vi "car coordinate move position in out.vi"(7 "Position in 2":T1, 8 "error in (no error)":errorcluster, 9 "Position in":T1, 11 "move":cluster{"X":dbl, "Y":dbl}) -> (0 "error out":errorcluster, 1 "Position out":T1)   [LabVIEW 2019]
uses:
  move/position cluster.ctl
  V A J control/move cluster(VAJ).ctl
panel:
  out "x+y":dbl
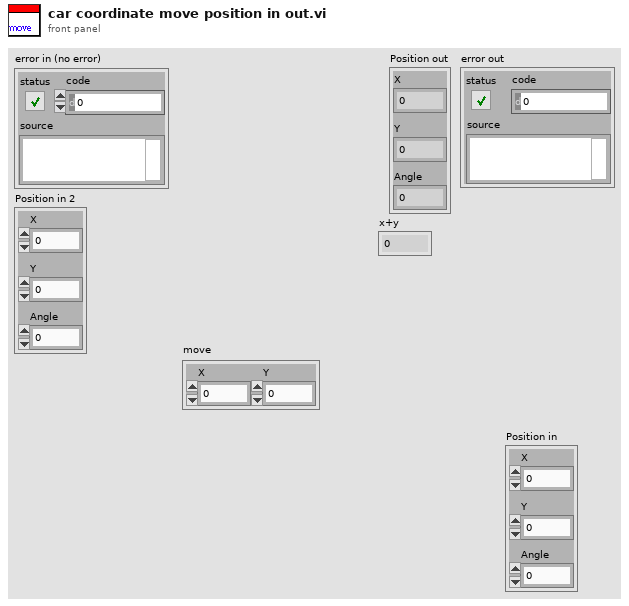
[diagram p1: front panel]
types:
  T1 = typedef "position cluster.ctl" = cluster{"X":dbl, "Y":dbl, "Angle":dbl}
  T2 = typedef "move cluster(VAJ).ctl" = cluster{"X":dbl, "Y":dbl, "degree":dbl, "other":string}
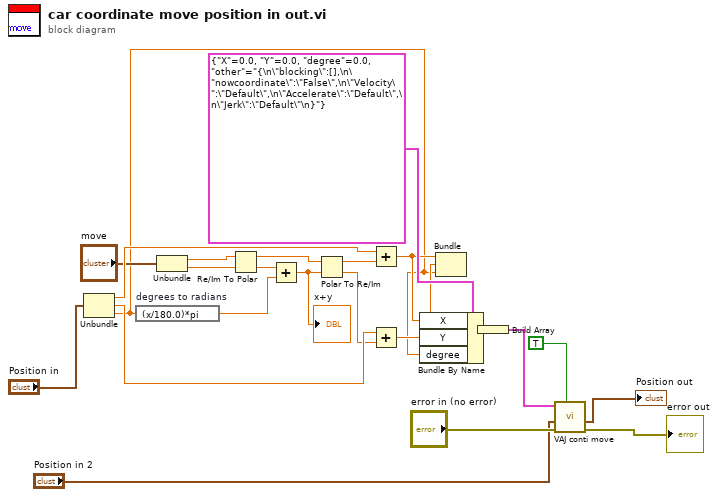
[diagram p0: block diagram]
diagram:
  n1 = Unbundle("Position in") -> ("X"=w19:dbl, "Y"=w18:dbl, "Angle"=w3:dbl)
  n2 = expression code="(x/180.0)*pi" "degrees to radians"(w3) -> (w23:dbl)
  n3 = Unbundle("move") -> ("X"=w14:dbl, "Y"=w13:dbl)
  n4 = Re/Im To Polar(2:w13, 3:w14) -> (0:w22:dbl, 1:w20:dbl)
  n5 = Add(x=w22, y=w23) -> (x+y=w21:dbl)
  "x+y" <- w21
  n6 = Polar To Re/Im(2:w21, 3:w20) -> (0:w16:dbl, 1:w17:dbl)
  n7 = Add(x=w19, y=w17) -> (x+y=w5:dbl)
  n8 = Add(x=w18, y=w16) -> (x+y=w4:dbl)
  n9 = Bundle By Name(cluster=T2 {"X"=0.0, "Y"=0.0, "degree"=0.0, "other"="{\n\"blocking\":[],\n\"nowcoordinate\":\"False\",\n\"Velocity\":\"Default\",\n\"Accelerate\":\"Default\",\n\"Jerk\":\"Default\"\n}"} ("move in"), "X"=w5, "Y"=w4, "degree"=w3) -> (w12:T2)
  n10 = Bundle(w5, w4, "Angle"=w3) -> ()  [unwired: 1 in, 1 out]
  n11 = Build Array(w12) -> (w11:T2[])
  n12 = call "VAJ conti move.vi"("move?"=TRUE, "error in (no error)"="error in (no error)", "Position in"="Position in 2", "move in"=w11) -> ("error out"=→"error out":errorcluster, "Position out"=→"Position out":T1)  [unwired: 5 in, 1 out]
